vi "Motor Speeds Global Variable.vi"(8 "Set?":bool, 11 "Motor Speeds":dbl[](array[numeric])) -> (3 "Motor Speeds out":dbl[](array[numeric]))   [LabVIEW 2013]
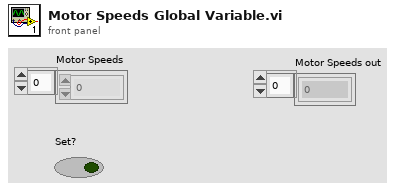
[diagram p1: front panel]
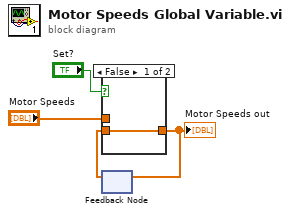
[diagram p0: block diagram]
diagram:
  n1 = feedback #1() -> (w2:dbl[])  [unwired: 1 in]
  n2 = case shown="False" "Set?" {
    tunnel: [w5 w6] -> w1
    tunnel: "Motor Speeds" -> [_ w6]
    tunnel: w2 -> [w5 _]
    frame False {
    }
    frame True {
    }
  }
  "Motor Speeds out" <- w1
  n3 = feedback-in #1(w1) -> ()
